vi "保存流程文件.vi"(8 "错误输入（无错误）":errorcluster, 11 "流程":T1 {"进样流程"."进样流程-进样"."步骤二："."功能" items=["加标", "进样", "排液", "搅拌", "定量", "延时"]; "进样流程"."进样流程-进样"."步骤一："."功能" items=["加标", "进样", "排液", "搅拌", "定量", "延时"]; "进样流程"."进样流程-进样"."步骤四："."功能" items=["加标", "进样", "排液", "搅拌", "定量", "延时"]; "进样流程"."进样流程-进样"."步骤三："."功能" items=["加标", "进样", "排液", "搅拌", "定量", "延时"]; "进样流程"."进样流程-进样"."步骤六："."功能" items=["加标", "进样", "排液", "搅拌", "定量", "延时"]; "进样流程"."进样流程-进样"."步骤五："."功能" items=["加标", "进样", "排液", "搅拌", "定量", "延时"]; "进样流程"."进样流程-进样"."步骤八："."功能" items=["加标", "进样", "排液", "搅拌", "定量", "延时"]; "进样流程"."进样流程-进样"."步骤七："."功能" items=["加标", "进样", "排液", "搅拌", "定量", "延时"]; "进样流程"."进样流程-进样"."步骤十："."功能" items=["加标", "进样", "排液", "搅拌", "定量", "延时"]; "进样流程"."进样流程-进样"."步骤九："."功能" items=["加标", "进样", "排液", "搅拌", "定量", "延时"]; "进样流程"."进样流程-润洗"."步骤二："."功能" items=["加标", "进样", "排液", "搅拌", "定量", "延时"]; "进样流程"."进样流程-润洗"."步骤一："."功能" items=["加标", "进样", "排液", "搅拌", "定量", "延时"]; "进样流程"."进样流程-润洗"."步骤四："."功能" items=["加标", "进样", "排液", "搅拌", "定量", "延时"]; "进样流程"."进样流程-润洗"."步骤三："."功能" items=["加标", "进样", "排液", "搅拌", "定量", "延时"]; "进样流程"."进样流程-润洗"."步骤六："."功能" items=["加标", "进样", "排液", "搅拌", "定量", "延时"]; "进样流程"."进样流程-润洗"."步骤五："."功能" items=["加标", "进样", "排液", "搅拌", "定量", "延时"]; "进样流程"."进样流程-润洗"."步骤八："."功能" items=["加标", "进样", "排液", "搅拌", "定量", "延时"]; "进样流程"."进样流程-润洗"."步骤七："."功能" items=["加标", "进样", "排液", "搅拌", "定量", "延时"]; "进样流程"."进样流程-润洗"."步骤十："."功能" items=["加标", "进样", "排液", "搅拌", "定量", "延时"]; "进样流程"."进样流程-润洗"."步骤九："."功能" items=["加标", "进样", "排液", "搅拌", "定量", "延时"]; "排液流程"."步骤二："."功能" items=["加标", "进样", "排液", "搅拌", "定量", "延时"]; "排液流程"."步骤一："."功能" items=["加标", "进样", "排液", "搅拌", "定量", "延时"]; "排液流程"."步骤四："."功能" items=["加标", "进样", "排液", "搅拌", "定量", "延时"]; "排液流程"."步骤三："."功能" items=["加标", "进样", "排液", "搅拌", "定量", "延时"]; "排液流程"."步骤六："."功能" items=["加标", "进样", "排液", "搅拌", "定量", "延时"]; "排液流程"."步骤五："."功能" items=["加标", "进样", "排液", "搅拌", "定量", "延时"]; "排液流程"."步骤八："."功能" items=["加标", "进样", "排液", "搅拌", "定量", "延时"]; "排液流程"."步骤七："."功能" items=["加标", "进样", "排液", "搅拌", "定量", "延时"]; "排液流程"."步骤十："."功能" items=["加标", "进样", "排液", "搅拌", "定量", "延时"]; "排液流程"."步骤九："."功能" items=["加标", "进样", "排液", "搅拌", "定量", "延时"]; "加标流程"."加标流程-加标"."步骤二："."功能" items=["加标", "进样", "排液", "搅拌", "定量", "延时"]; "加标流程"."加标流程-加标"."步骤一："."功能" items=["加标", "进样", "排液", "搅拌", "定量", "延时"]; "加标流程"."加标流程-加标"."步骤四："."功能" items=["加标", "进样", "排液", "搅拌", "定量", "延时"]; "加标流程"."加标流程-加标"."步骤三："."功能" items=["加标", "进样", "排液", "搅拌", "定量", "延时"]; "加标流程"."加标流程-加标"."步骤六："."功能" items=["加标", "进样", "排液", "搅拌", "定量", "延时"]; "加标流程"."加标流程-加标"."步骤五："."功能" items=["加标", "进样", "排液", "搅拌", "定量", "延时"]; "加标流程"."加标流程-加标"."步骤八："."功能" items=["加标", "进样", "排液", "搅拌", "定量", "延时"]; "加标流程"."加标流程-加标"."步骤七："."功能" items=["加标", "进样", "排液", "搅拌", "定量", "延时"]; "加标流程"."加标流程-加标"."步骤十："."功能" items=["加标", "进样", "排液", "搅拌", "定量", "延时"]; "加标流程"."加标流程-加标"."步骤九："."功能" items=["加标", "进样", "排液", "搅拌", "定量", "延时"]; "加标流程"."加标流程-定量"."步骤二："."功能" items=["加标", "进样", "排液", "搅拌", "定量", "延时"]; "加标流程"."加标流程-定量"."步骤一："."功能" items=["加标", "进样", "排液", "搅拌", "定量", "延时"]; "加标流程"."加标流程-定量"."步骤四："."功能" items=["加标", "进样", "排液", "搅拌", "定量", "延时"]; "加标流程"."加标流程-定量"."步骤三："."功能" items=["加标", "进样", "排液", "搅拌", "定量", "延时"]; "加标流程"."加标流程-定量"."步骤六："."功能" items=["加标", "进样", "排液", "搅拌", "定量", "延时"]; "加标流程"."加标流程-定量"."步骤五："."功能" items=["加标", "进样", "排液", "搅拌", "定量", "延时"]; "加标流程"."加标流程-定量"."步骤八："."功能" items=["加标", "进样", "排液", "搅拌", "定量", "延时"]; "加标流程"."加标流程-定量"."步骤七："."功能" items=["加标", "进样", "排液", "搅拌", "定量", "延时"]; "加标流程"."加标流程-定量"."步骤十："."功能" items=["加标", "进样", "排液", "搅拌", "定量", "延时"]; "加标流程"."加标流程-定量"."步骤九："."功能" items=["加标", "进样", "排液", "搅拌", "定量", "延时"]; "加标流程"."加标流程-进样"."步骤二："."功能" items=["加标", "进样", "排液", "搅拌", "定量", "延时"]; "加标流程"."加标流程-进样"."步骤一："."功能" items=["加标", "进样", "排液", "搅拌", "定量", "延时"]; "加标流程"."加标流程-进样"."步骤四："."功能" items=["加标", "进样", "排液", "搅拌", "定量", "延时"]; "加标流程"."加标流程-进样"."步骤三："."功能" items=["加标", "进样", "排液", "搅拌", "定量", "延时"]; "加标流程"."加标流程-进样"."步骤六："."功能" items=["加标", "进样", "排液", "搅拌", "定量", "延时"]; "加标流程"."加标流程-进样"."步骤五："."功能" items=["加标", "进样", "排液", "搅拌", "定量", "延时"]; "加标流程"."加标流程-进样"."步骤八："."功能" items=["加标", "进样", "排液", "搅拌", "定量", "延时"]; "加标流程"."加标流程-进样"."步骤七："."功能" items=["加标", "进样", "排液", "搅拌", "定量", "延时"]; "加标流程"."加标流程-进样"."步骤十："."功能" items=["加标", "进样", "排液", "搅拌", "定量", "延时"]; "加标流程"."加标流程-进样"."步骤九："."功能" items=["加标", "进样", "排液", "搅拌", "定量", "延时"]; "加标流程"."加标流程-润洗"."步骤二："."功能" items=["加标", "进样", "排液", "搅拌", "定量", "延时"]; "加标流程"."加标流程-润洗"."步骤一："."功能" items=["加标", "进样", "排液", "搅拌", "定量", "延时"]; "加标流程"."加标流程-润洗"."步骤四："."功能" items=["加标", "进样", "排液", "搅拌", "定量", "延时"]; "加标流程"."加标流程-润洗"."步骤三："."功能" items=["加标", "进样", "排液", "搅拌", "定量", "延时"]; "加标流程"."加标流程-润洗"."步骤六："."功能" items=["加标", "进样", "排液", "搅拌", "定量", "延时"]; "加标流程"."加标流程-润洗"."步骤五："."功能" items=["加标", "进样", "排液", "搅拌", "定量", "延时"]; "加标流程"."加标流程-润洗"."步骤八："."功能" items=["加标", "进样", "排液", "搅拌", "定量", "延时"]; "加标流程"."加标流程-润洗"."步骤七："."功能" items=["加标", "进样", "排液", "搅拌", "定量", "延时"]; "加标流程"."加标流程-润洗"."步骤十："."功能" items=["加标", "进样", "排液", "搅拌", "定量", "延时"]; "加标流程"."加标流程-润洗"."步骤九："."功能" items=["加标", "进样", "排液", "搅拌", "定量", "延时"]; "加标润洗流程"."步骤二："."功能" items=["加标", "进样", "排液", "搅拌", "定量", "延时"]; "加标润洗流程"."步骤一："."功能" items=["加标", "进样", "排液", "搅拌", "定量", "延时"]; "加标润洗流程"."步骤四："."功能" items=["加标", "进样", "排液", "搅拌", "定量", "延时"]; "加标润洗流程"."步骤三："."功能" items=["加标", "进样", "排液", "搅拌", "定量", "延时"]; "加标润洗流程"."步骤六："."功能" items=["加标", "进样", "排液", "搅拌", "定量", "延时"]; "加标润洗流程"."步骤五："."功能" items=["加标", "进样", "排液", "搅拌", "定量", "延时"]; "加标润洗流程"."步骤八："."功能" items=["加标", "进样", "排液", "搅拌", "定量", "延时"]; "加标润洗流程"."步骤七："."功能" items=["加标", "进样", "排液", "搅拌", "定量", "延时"]; "加标润洗流程"."步骤十："."功能" items=["加标", "进样", "排液", "搅拌", "定量", "延时"]; "加标润洗流程"."步骤九："."功能" items=["加标", "进样", "排液", "搅拌", "定量", "延时"]; "水样润洗流程"."步骤二："."功能" items=["加标", "进样", "排液", "搅拌", "定量", "延时"]; "水样润洗流程"."步骤一："."功能" items=["加标", "进样", "排液", "搅拌", "定量", "延时"]; "水样润洗流程"."步骤四："."功能" items=["加标", "进样", "排液", "搅拌", "定量", "延时"]; "水样润洗流程"."步骤三："."功能" items=["加标", "进样", "排液", "搅拌", "定量", "延时"]; "水样润洗流程"."步骤六："."功能" items=["加标", "进样", "排液", "搅拌", "定量", "延时"]; "水样润洗流程"."步骤五："."功能" items=["加标", "进样", "排液", "搅拌", "定量", "延时"]; "水样润洗流程"."步骤八："."功能" items=["加标", "进样", "排液", "搅拌", "定量", "延时"]; "水样润洗流程"."步骤七："."功能" items=["加标", "进样", "排液", "搅拌", "定量", "延时"]; "水样润洗流程"."步骤十："."功能" items=["加标", "进样", "排液", "搅拌", "定量", "延时"]; "水样润洗流程"."步骤九："."功能" items=["加标", "进样", "排液", "搅拌", "定量", "延时"]}) -> (0 "错误输出":errorcluster, 3 "cancelled":bool caption="取消")   [LabVIEW 2016, in "质控单元V4.lvlib"]
panel:
  out "JSON字符串":string
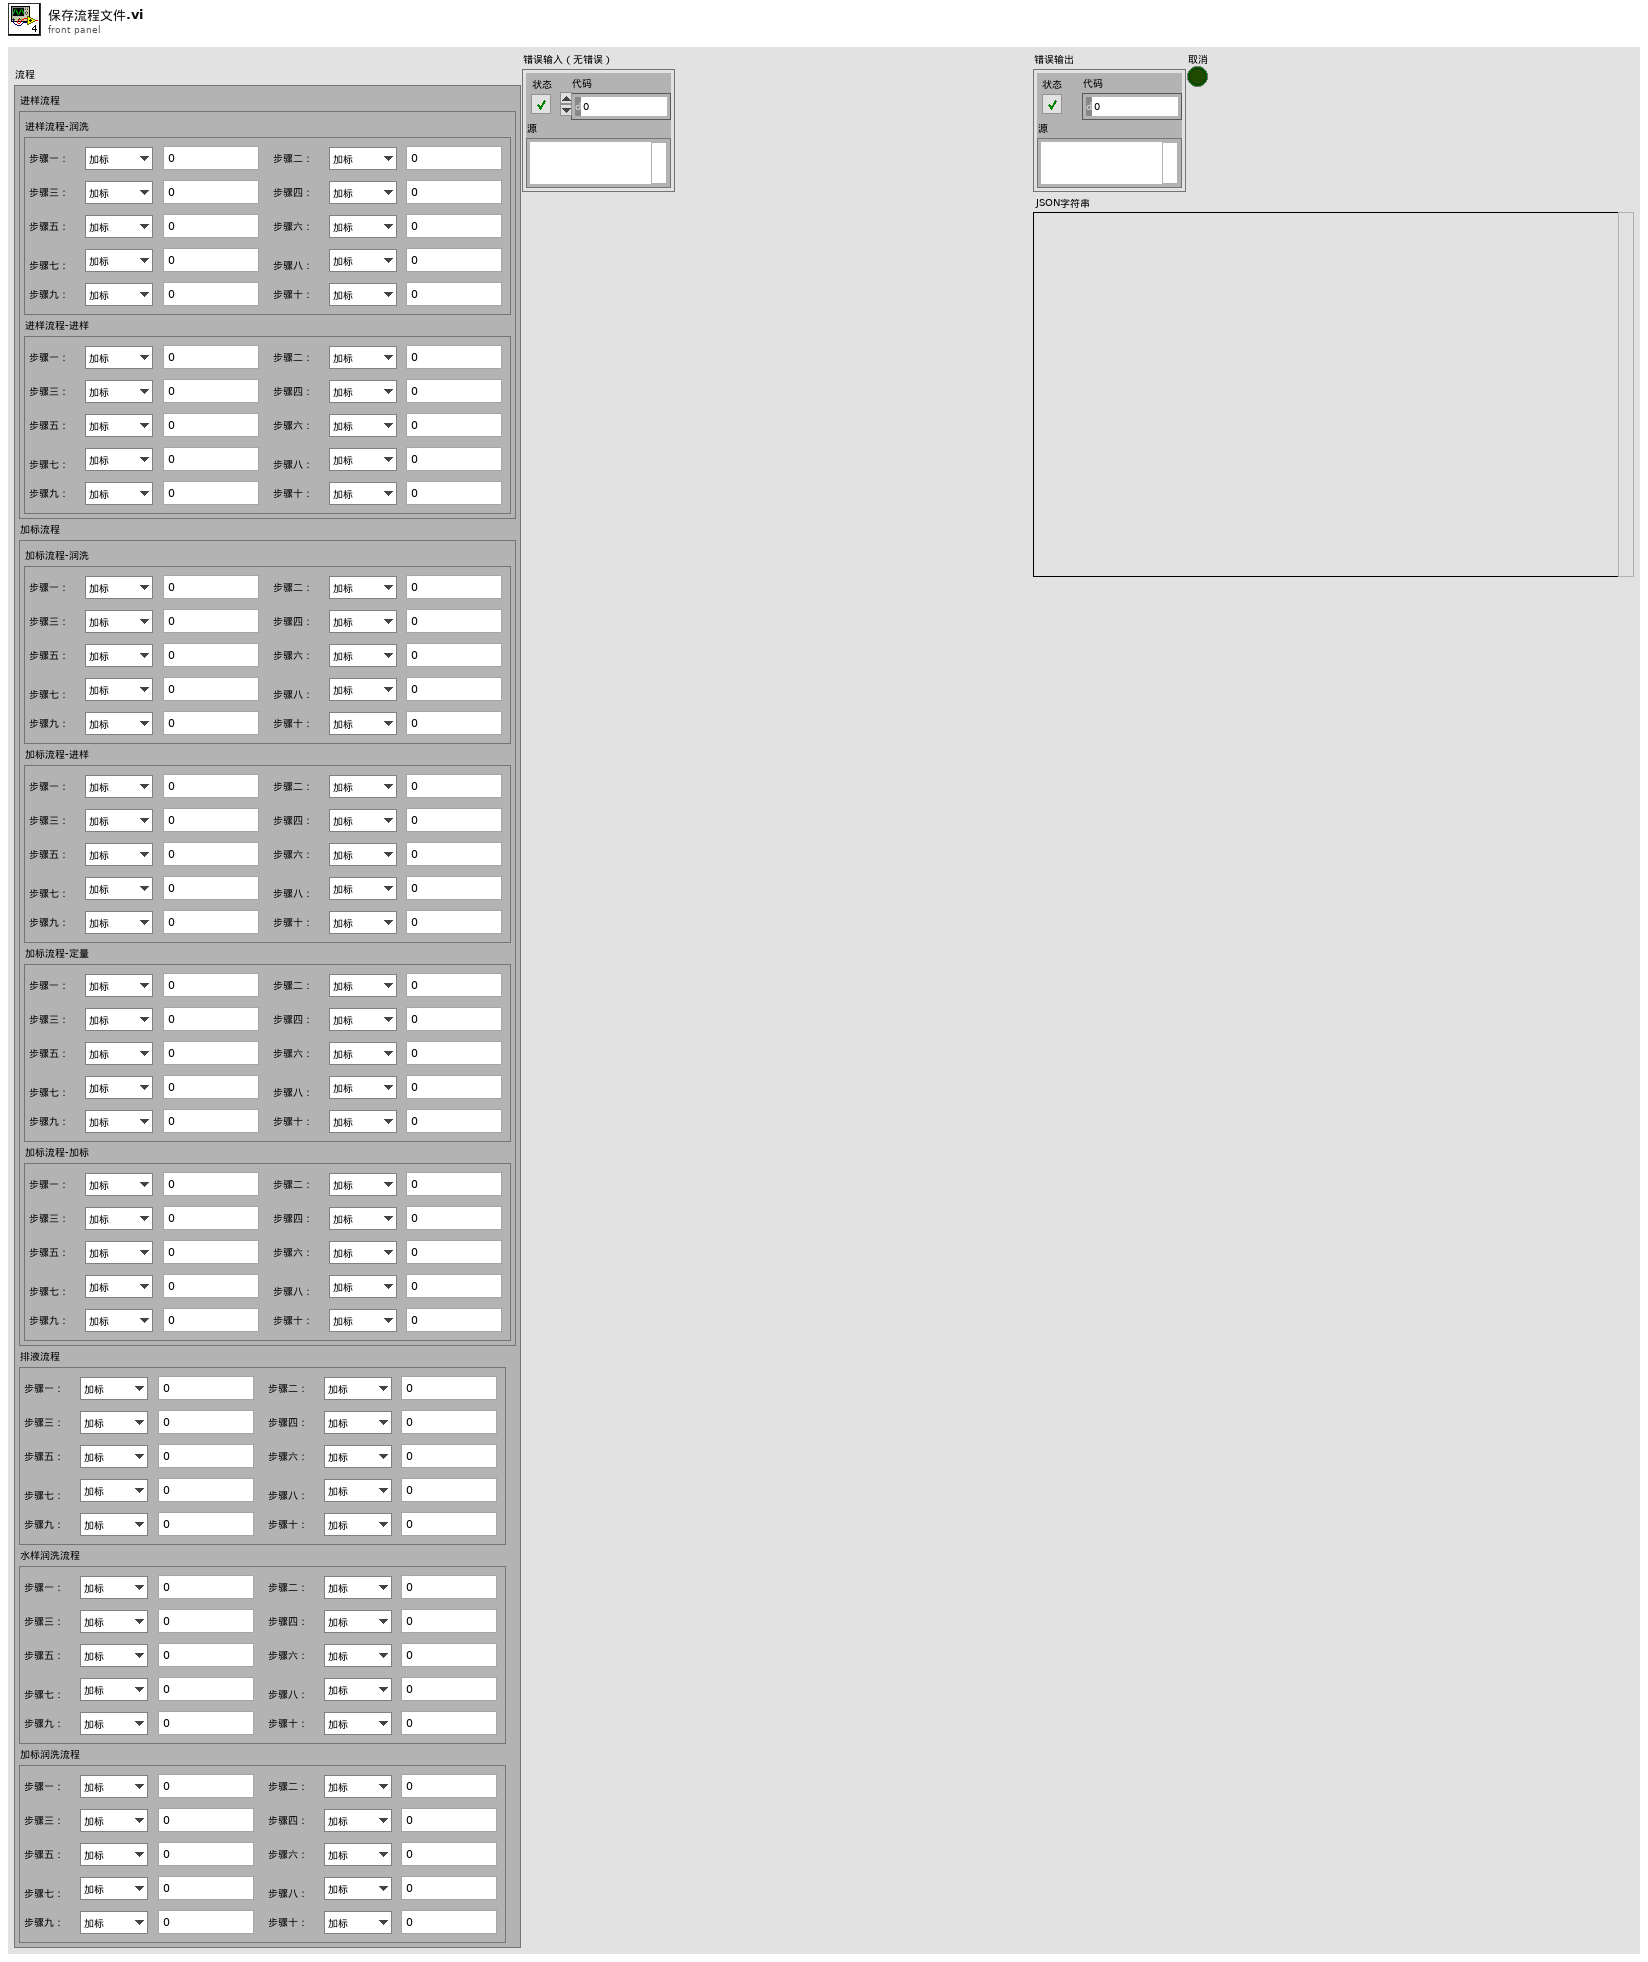
[diagram p1: front panel]
types:
  T1 = cluster{"进样流程":cluster{"进样流程-润洗":cluster{"步骤一：":cluster{"功能":u16, "值":sgl}, "步骤二：":cluster{"功能":u16, "值":sgl}, "步骤三：":cluster{"功能":u16, "值":sgl}, "步骤四：":cluster{"功能":u16, "值":sgl}, "步骤五：":cluster{"功能":u16, "值":sgl}, "步骤六：":cluster{"功能":u16, "值":sgl}, "步骤七：":cluster{"功能":u16, "值":sgl}, "步骤八：":cluster{"功能":u16, "值":sgl}, "步骤九：":cluster{"功能":u16, "值":sgl}, "步骤十：":cluster{"功能":u16, "值":sgl}}, "进样流程-进样":cluster{"步骤一：":cluster{"功能":u16, "值":sgl}, "步骤二：":cluster{"功能":u16, "值":sgl}, "步骤三：":cluster{"功能":u16, "值":sgl}, "步骤四：":cluster{"功能":u16, "值":sgl}, "步骤五：":cluster{"功能":u16, "值":sgl}, "步骤六：":cluster{"功能":u16, "值":sgl}, "步骤七：":cluster{"功能":u16, "值":sgl}, "步骤八：":cluster{"功能":u16, "值":sgl}, "步骤九：":cluster{"功能":u16, "值":sgl}, "步骤十：":cluster{"功能":u16, "值":sgl}}}, "加标流程":cluster{"加标流程-润洗":cluster{"步骤一：":cluster{"功能":u16, "值":sgl}, "步骤二：":cluster{"功能":u16, "值":sgl}, "步骤三：":cluster{"功能":u16, "值":sgl}, "步骤四：":cluster{"功能":u16, "值":sgl}, "步骤五：":cluster{"功能":u16, "值":sgl}, "步骤六：":cluster{"功能":u16, "值":sgl}, "步骤七：":cluster{"功能":u16, "值":sgl}, "步骤八：":cluster{"功能":u16, "值":sgl}, "步骤九：":cluster{"功能":u16, "值":sgl}, "步骤十：":cluster{"功能":u16, "值":sgl}}, "加标流程-进样":cluster{"步骤一：":cluster{"功能":u16, "值":sgl}, "步骤二：":cluster{"功能":u16, "值":sgl}, "步骤三：":cluster{"功能":u16, "值":sgl}, "步骤四：":cluster{"功能":u16, "值":sgl}, "步骤五：":cluster{"功能":u16, "值":sgl}, "步骤六：":cluster{"功能":u16, "值":sgl}, "步骤七：":cluster{"功能":u16, "值":sgl}, "步骤八：":cluster{"功能":u16, "值":sgl}, "步骤九：":cluster{"功能":u16, "值":sgl}, "步骤十：":cluster{"功能":u16, "值":sgl}}, "加标流程-定量":cluster{"步骤一：":cluster{"功能":u16, "值":sgl}, "步骤二：":cluster{"功能":u16, "值":sgl}, "步骤三：":cluster{"功能":u16, "值":sgl}, "步骤四：":cluster{"功能":u16, "值":sgl}, "步骤五：":cluster{"功能":u16, "值":sgl}, "步骤六：":cluster{"功能":u16, "值":sgl}, "步骤七：":cluster{"功能":u16, "值":sgl}, "步骤八：":cluster{"功能":u16, "值":sgl}, "步骤九：":cluster{"功能":u16, "值":sgl}, "步骤十：":cluster{"功能":u16, "值":sgl}}, "加标流程-加标":cluster{"步骤一：":cluster{"功能":u16, "值":sgl}, "步骤二：":cluster{"功能":u16, "值":sgl}, "步骤三：":cluster{"功能":u16, "值":sgl}, "步骤四：":cluster{"功能":u16, "值":sgl}, "步骤五：":cluster{"功能":u16, "值":sgl}, "步骤六：":cluster{"功能":u16, "值":sgl}, "步骤七：":cluster{"功能":u16, "值":sgl}, "步骤八：":cluster{"功能":u16, "值":sgl}, "步骤九：":cluster{"功能":u16, "值":sgl}, "步骤十：":cluster{"功能":u16, "值":sgl}}}, "排液流程":cluster{"步骤一：":cluster{"功能":u16, "值":sgl}, "步骤二：":cluster{"功能":u16, "值":sgl}, "步骤三：":cluster{"功能":u16, "值":sgl}, "步骤四：":cluster{"功能":u16, "值":sgl}, "步骤五：":cluster{"功能":u16, "值":sgl}, "步骤六：":cluster{"功能":u16, "值":sgl}, "步骤七：":cluster{"功能":u16, "值":sgl}, "步骤八：":cluster{"功能":u16, "值":sgl}, "步骤九：":cluster{"功能":u16, "值":sgl}, "步骤十：":cluster{"功能":u16, "值":sgl}}, "水样润洗流程":cluster{"步骤一：":cluster{"功能":u16, "值":sgl}, "步骤二：":cluster{"功能":u16, "值":sgl}, "步骤三：":cluster{"功能":u16, "值":sgl}, "步骤四：":cluster{"功能":u16, "值":sgl}, "步骤五：":cluster{"功能":u16, "值":sgl}, "步骤六：":cluster{"功能":u16, "值":sgl}, "步骤七：":cluster{"功能":u16, "值":sgl}, "步骤八：":cluster{"功能":u16, "值":sgl}, "步骤九：":cluster{"功能":u16, "值":sgl}, "步骤十：":cluster{"功能":u16, "值":sgl}}, "加标润洗流程":cluster{"步骤一：":cluster{"功能":u16, "值":sgl}, "步骤二：":cluster{"功能":u16, "值":sgl}, "步骤三：":cluster{"功能":u16, "值":sgl}, "步骤四：":cluster{"功能":u16, "值":sgl}, "步骤五：":cluster{"功能":u16, "值":sgl}, "步骤六：":cluster{"功能":u16, "值":sgl}, "步骤七：":cluster{"功能":u16, "值":sgl}, "步骤八：":cluster{"功能":u16, "值":sgl}, "步骤九：":cluster{"功能":u16, "值":sgl}, "步骤十：":cluster{"功能":u16, "值":sgl}}}
  T2 = cluster{"flow1":cluster{"Type":u16, "Value":sgl}[], "flow2":cluster{"Type":u16, "Value":sgl}[], "flow3":cluster{"Type":u16, "Value":sgl}[], "flow4":cluster{"Type":u16, "Value":sgl}[], "flow5":cluster{"Type":u16, "Value":sgl}[]}
  T3 = cluster{"步骤一：":cluster{"功能":u16, "值":sgl}, "步骤二：":cluster{"功能":u16, "值":sgl}, "步骤三：":cluster{"功能":u16, "值":sgl}, "步骤四：":cluster{"功能":u16, "值":sgl}, "步骤五：":cluster{"功能":u16, "值":sgl}, "步骤六：":cluster{"功能":u16, "值":sgl}, "步骤七：":cluster{"功能":u16, "值":sgl}, "步骤八：":cluster{"功能":u16, "值":sgl}, "步骤九：":cluster{"功能":u16, "值":sgl}, "步骤十：":cluster{"功能":u16, "值":sgl}}
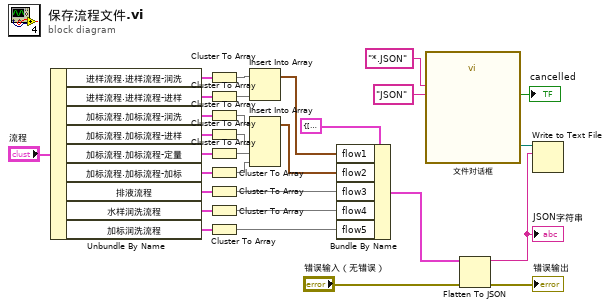
[diagram p0: block diagram]
diagram:
  n1 = Unbundle By Name("流程") -> ("进样流程.进样流程-润洗"=w27:T3, "进样流程.进样流程-进样"=w26:T3, "加标流程.加标流程-润洗"=w20:T3, "加标流程.加标流程-进样"=w19:T3, "加标流程.加标流程-定量"=w18:T3, "加标流程.加标流程-加标"=w17:T3, "排液流程"=w14:T3, "水样润洗流程"=w13:T3, "加标润洗流程"=w12:T3)
  n2 = Cluster To Array(cluster=w27) -> (array=w25:cluster{"功能":u16, "值":sgl}[])
  n3 = Cluster To Array(cluster=w26) -> (array=w24:cluster{"功能":u16, "值":sgl}[])
  n4 = Cluster To Array(cluster=w20) -> (array=w21:cluster{"功能":u16, "值":sgl}[])
  n5 = Cluster To Array(cluster=w19) -> (array=w22:cluster{"功能":u16, "值":sgl}[])
  n6 = Cluster To Array(cluster=w18) -> (array=w16:cluster{"功能":u16, "值":sgl}[])
  n7 = Cluster To Array(cluster=w17) -> (array=w15:cluster{"功能":u16, "值":sgl}[])
  n8 = Cluster To Array(cluster=w14) -> (array=w10:cluster{"功能":u16, "值":sgl}[])
  n9 = Cluster To Array(cluster=w13) -> (array=w9:cluster{"功能":u16, "值":sgl}[])
  n10 = Cluster To Array(cluster=w12) -> (array=w8:cluster{"功能":u16, "值":sgl}[])
  n11 = Insert Into Array(array=w25, new element=w24) -> (w23:cluster{"功能":u16, "值":sgl}[])  [unwired: 1 in]
  n12 = Insert Into Array(array=w21, new element #1=w22, new element #2=w16, new element #3=w15) -> (w11:cluster{"功能":u16, "值":sgl}[])  [unwired: 1 in]
  n13 = Bundle By Name(cluster=T2 {"flow1"=[], "flow2"=[], "flow3"=[], "flow4"=[], "flow5"=[]}, "flow1"=w23, "flow2"=w11, "flow3"=w10, "flow4"=w9, "flow5"=w8) -> (w28:T2)
  n14 = call "文件对话框"("pattern (all files)"="*.JSON" ("pattern label"), "pattern label"="JSON") -> ("selected path"=w4:path, "cancelled"=→"cancelled":bool)  [unwired: 10 in, 2 out]
  n15 = Flatten To JSON(anything=w28, error in (no error)="错误输入（无错误）") -> (JSON string=w5:string, 11:→"错误输出":errorcluster)  [unwired: 1 in]
  "JSON字符串" <- w5
  n16 = Write to Text File(file (use dialog)=w4, text=w5) -> ()  [unwired: 2 in, 3 out]
